vi "runSingleDPScriptV2.vi"(6 "HWLoop?":bool, 8 "error in (no error)":errorcluster, 9 "index":i32, 10 "status in":refnum<vi>, 11 "ExperimentRunner in":refnum<class "ExperimentRunner.lvclass">) -> (0 "error out":errorcluster, 2 "status out":refnum<vi>, 3 "ExperimentRunner out":refnum<class "ExperimentRunner.lvclass">)   [LabVIEW 2009, in "Views.lvlib" / "ExperimentControl.lvlib" / "ExperimentRunner.lvclass"]
doc: "Run a single script"
uses:
  ExperimentRunner.lvclass
  ExperimentRunner.lvclass/ExperimentRunner.ctl
  Hal/HWController/HWControllerEvents/HWControllerEvents.lvclass
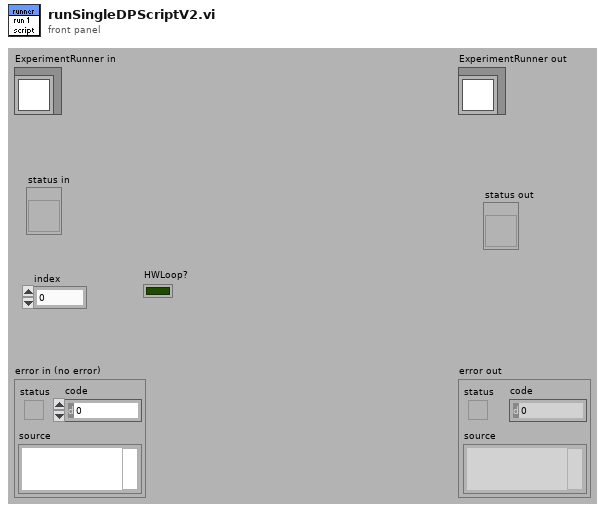
[diagram p1: front panel]
types:
  T1 = enum16{"start", "stop", "statusInquiry", "configure", "resetError", "resourcesInquiry", "reserveResources", "initialise", "resetAllChannels", "staticUpdate", "close", "HWStatus", "error", "resourcesAvailable", "resourcesReserved", "compilerError", "compiledScript", "compilingScript", "runScript", "configureCompiledScript"}
  T2 = enum16{"Ready", "Compiling", "Configured", "Running", "Stopping", "Unresolved Error"}
  T3 = cluster{"incomingEventTypes":cluster{"start":cluster{"Boolean":bool}, "stop":cluster{"Boolean":bool}, "statusInquiry":cluster{"Boolean":bool}, "configure":cluster{"DPScriptPath":path, "TimeStamp":string, "HWLoop?":bool}, "resetError":cluster{"Boolean":bool}, "resourcesInquiry":cluster{"Boolean":bool}, "reserveResources":cluster{"HWList":string[]}, "initialise":cluster{"HWList":string[]}, "close":cluster{"Boolean":bool}, "resetAllChannels":cluster{"Boolean":bool}, "staticChannelUpdate":cluster{"channel_address":string, "calibratedValue":dbl}, "runScript":cluster{"DPScriptPath":path, "TimeStamp":string, "HWLoop?":bool}, "compilingScript":cluster{"Path":path}, "compiledScript":cluster{"Path":path, "timeCompileAt":string}, "compilerError":cluster{"Path":path}, "configureCompiledScript":cluster{"DPScriptPath":path, "TimeStamp":string, "HWLoop?":bool, "CompiledScript":cluster{"ScriptListCompiler.lvclass":refnum<class "ScriptListCompiler.lvclass">, "aoChannels":refnum<class "AnalogOutput.lvclass">[], "doChannels":refnum<class "DigitalOutput.lvclass">[], "rfChannels":refnum<class "DDSOutput.lvclass">[]}}, "restartCompiler":cluster{"restart":bool}, "staticRfChannelUpdate":cluster{"channel_address":string, "Output":cluster{"Frequency(MHz)":dbl, "Amplitude":dbl, "Phase":dbl, "OutputForm":enum16{"Sine", "Square", "Triangle", "Arbitrary"}}}}, "outgoingEventTypes":cluster{"HWStatus":cluster{"status":enum16{"Ready", "Compiling", "Configured", "Running", "Stopping", "Unresolved Error"}}, "error":cluster{"error out":errorcluster}, "resourcesAvailable":cluster{"availableHWList":string[], "reservedHWList":string[]}, "resourcesReserved":cluster{"reservedHWList":string[]}}}
  T4 = cluster{"DPScriptPath":path, "TimeStamp":string, "HWLoop?":bool}
  T5 = cluster{"eventId":enum16{"start", "stop", "statusInquiry", "configure", "resetError", "resourcesInquiry", "reserveResources", "initialise", "resetAllChannels", "staticUpdate", "close", "HWStatus", "error", "resourcesAvailable", "resourcesReserved", "compilerError", "compiledScript", "compilingScript", "runScript", "configureCompiledScript"}, "runScript":cluster{"DPScriptPath":path, "TimeStamp":string, "HWLoop?":bool}}
  T6 = cluster{"eventId":enum16{"start", "stop", "statusInquiry", "configure", "resetError", "resourcesInquiry", "reserveResources", "initialise", "resetAllChannels", "staticUpdate", "close", "HWStatus", "error", "resourcesAvailable", "resourcesReserved", "compilerError", "compiledScript", "compilingScript", "runScript", "configureCompiledScript"}, "start":cluster{"Boolean":bool}}
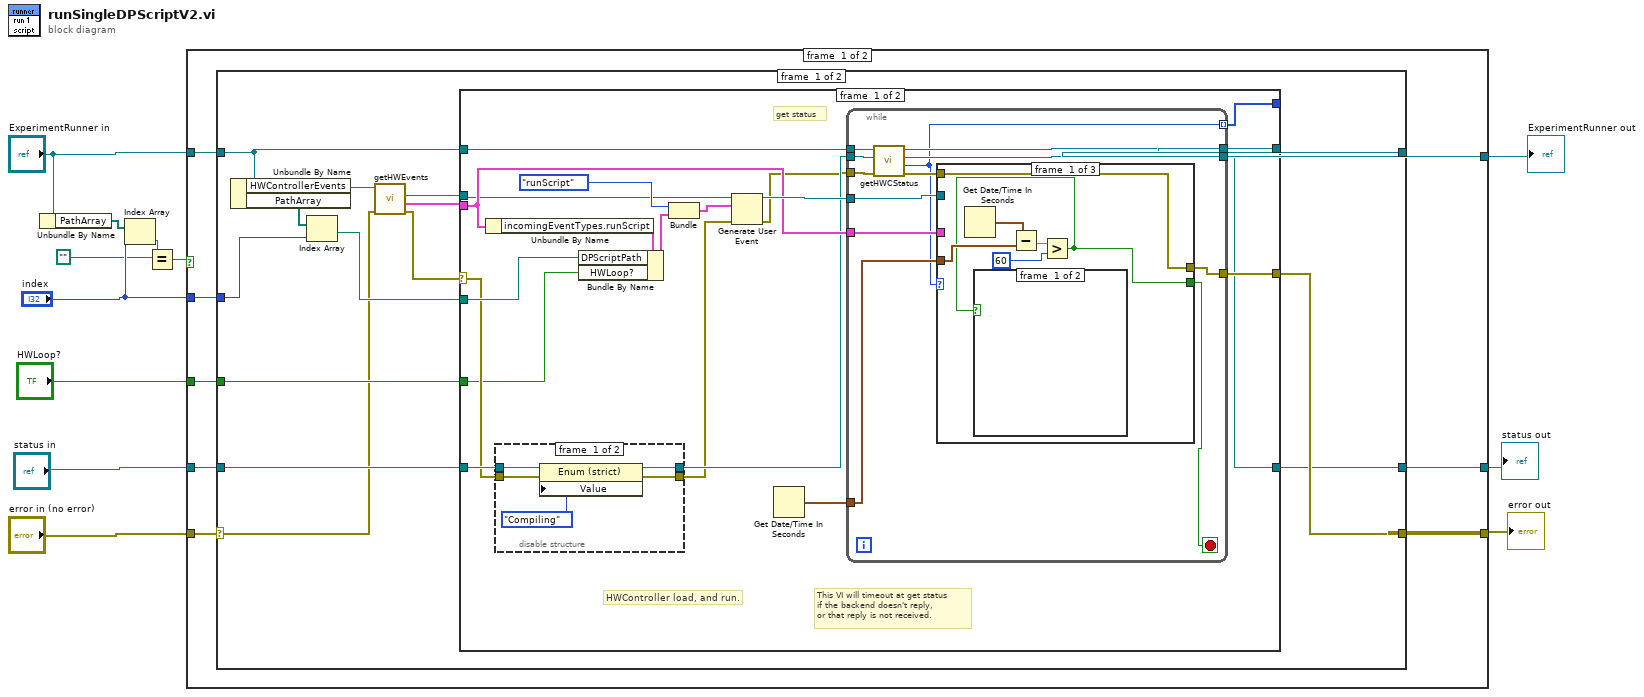
[diagram p0: block diagram]
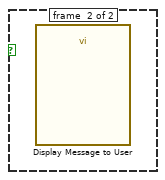
[diagram p3: hidden frame]
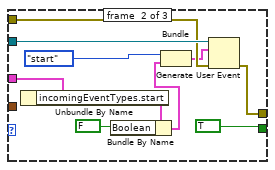
[diagram p4: hidden frame]
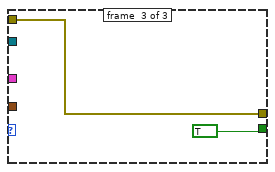
[diagram p5: hidden frame]
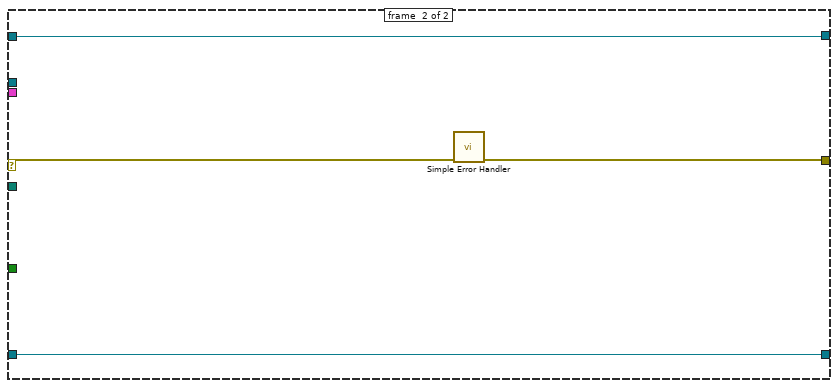
[diagram p6: hidden frame]
diagram:
  n1 = Unbundle By Name("ExperimentRunner in") -> ("PathArray"=w7:path[])
  n2 = Index Array(array=w7, index="index") -> (element=w5:path)
  n3 = Equal?(x=w5, y=path "") -> (x = y?=w3:bool)
  n4 = case shown="False" w3 {
    tunnel: "error in (no error)" -> [w20 w99]
    tunnel: [w19 w99] -> w11
    tunnel: [w18 w101] -> w10
    tunnel: "status in" -> [w17 w100]
    tunnel: [w16 w100] -> w9
    tunnel: "ExperimentRunner in" -> [w15 w101]
    tunnel: "index" -> [w14 _]
    tunnel: "HWLoop?" -> [w13 _]
    frame #0 {
      n5 = case shown="No Error" w20 {
        selector: w20 -> [w21 w98]
        tunnel: [w32 w98] -> w19
        tunnel: [w25 w97] -> w18
        tunnel: w15 -> [w28 w97]
        tunnel: w14 -> [w33 _]
        tunnel: w17 -> [w27 w96]
        tunnel: [w26 w96] -> w16
        tunnel: w13 -> [w23 _]
        frame #0 {
          n6 = Unbundle By Name(w28) -> ("HWControllerEvents"=w31:refnum<class "HWControllerEvents.lvclass">, "PathArray"=w34:path[])
          n7 = Index Array(array=w34, index=w33) -> (element=w22:path)
          n8 = call-dynamic "getHWEvents.vi"("error in (no error)"=w21, "HWControllerEvents in"=w31) -> ("error out"=w24:errorcluster, "eventDataTypes"=w29:T3, "HWCEvent"=w30:refnum<user-event>)  [unwired: 6 in, 1 out]
          n9 = case shown="No Error" w24 {
            selector: w24 -> [w44 w95]
            tunnel: [w36 w94] -> w32
            tunnel: w30 -> [w41 _]
            tunnel: w29 -> [w50 _]
            tunnel: w22 -> [w53 _]
            tunnel: w28 -> [w49 w93]
            tunnel: [w37 w93] -> w25
            tunnel: w27 -> [w47 w92]
            tunnel: [w35 w92] -> w26
            tunnel: w23 -> [w43 _]
            tunnel: [w38 _] -> _
            frame #0 {
              # "This VI will timeout at get status\nif the backend doesn't reply,\nor that reply is not received."
              # "get status"
              # "HWController load, and run."
              n10 = Unbundle By Name(w50) -> ("incomingEventTypes.runScript"=w54:T4)
              n11 = disable-structure shown="Enabled" {
                disable-tunnel: w47 -> [w59 w61]
                disable-tunnel: [w58 w61] -> w46
                disable-tunnel: [w56 w60] -> w45
                disable-tunnel: w44 -> [w55 w60]
                frame #0 {
                  n12 = property class="Enum (strict)"(reference=w59, error in=w55, "Value"=T2."Compiling") -> (reference out=w58:refnum<vi>, error out=w56:errorcluster)
                }
                frame #1 {
                }
              }
              n13 = Bundle By Name(cluster=w54, "DPScriptPath"=w53, "HWLoop?"=w43) -> (w52:T4)
              n14 = Bundle("eventId"=T1."runScript", "runScript"=w52) -> (w40:T5)  [unwired: 1 in]
              n15 = Generate User Event(user event=w41, event data cluster=w40, error in=w45) -> (user event out=w51:refnum<user-event>, error out=w39:errorcluster)
              n16 = Get Date/Time In Seconds() -> (seconds since 1Jan1904=w48:timestamp)
              n17 = while {
                tunnel: w51 -> [w73]
                tunnel: w50 -> [w72]
                tunnel: [w71] -> w36
                tunnel: w39 -> [w70]
                tunnel: [w68] -> w37
                tunnel: w49 -> [w67]
                tunnel: w46 -> [w66]
                tunnel: [w65] -> w35
                tunnel: w48 -> [w64]
                tunnel: [w62] -> w38 mode=indexing
                stop <- w63 stop-if-true
                n18 = call "getHWCStatus.vi"("error in (no error)"=w70, "status in"=w66, "ExperimentRunner in"=w67) -> ("error out"=w69:errorcluster, "status"=w62:T2, "status out"=w65:refnum<vi>, "ExperimentRunner out"=w68:refnum<class "ExperimentRunner.lvclass">)  [unwired: 5 in]
                n19 = case shown="\"Configured\"" w62 {
                  tunnel: w73 -> [_ w89 _]
                  tunnel: w72 -> [_ w88 _]
                  tunnel: [w79 w87 w90] -> w71
                  tunnel: w69 -> [w79 w86 w90]
                  tunnel: [w74 TRUE TRUE] -> w63
                  tunnel: w64 -> [w77 _ _]
                  frame #0 {
                    n20 = Get Date/Time In Seconds() -> (seconds since 1Jan1904=w78:timestamp)
                    n21 = Subtract(x=w78, y=w77) -> (x-y=w76:dbl)
                    n22 = Greater?(x=w76, y=60) -> (0:w74:bool)
                    n23 = case shown="True" w74 {
                      frame #0 {
                      }
                      frame #1 {
                        n24 = call "Display Message to User"() -> ()  [unwired: 10 in, 2 out]
                      }
                    }
                  }
                  frame #1 {
                    n25 = Unbundle By Name(w88) -> ("incomingEventTypes.start"=w84:cluster{"Boolean":bool})
                    n26 = Bundle By Name(cluster=w84, "Boolean"=FALSE) -> (w83:cluster{"Boolean":bool})
                    n27 = Bundle("eventId"=T1."start", "start"=w83) -> (w85:T6)  [unwired: 1 in]
                    n28 = Generate User Event(user event=w89, event data cluster=w85, error in=w86) -> (error out=w87:errorcluster)  [unwired: 1 out]
                  }
                  frame #2 {
                  }
                }
              }
            }
            frame #1 {
              n29 = call <vilib>:"Simple Error Handler.vi"("error in (no error)"=w95) -> ("error out"=w94:errorcluster)  [unwired: 4 in, 4 out]
            }
          }
        }
        frame #1 {
        }
      }
    }
    frame #1 {
    }
  }
  "error out" <- w11
  "ExperimentRunner out" <- w10
  "status out" <- w9
